vi "Get Common Path.vi"(9 "Root Path":path, 11 "Target Path":path) -> (2 "Paths Equal":bool, 3 "Relative Path":path)   [LabVIEW 2019, in "MD Generator.lvlib"]
uses:
  MD Generator.lvlib
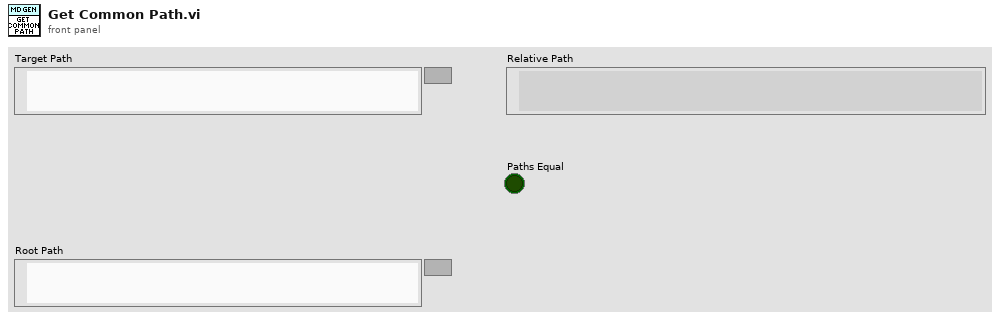
[diagram p1: front panel]
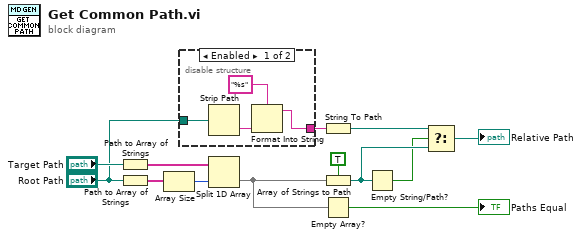
[diagram p0: block diagram]
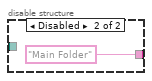
[diagram p2: hidden frame]
diagram:
  n1 = Path to Array of Strings(0:"Target Path") -> (2:w9:string[])  [unwired: 1 out]
  n2 = Path to Array of Strings(0:"Root Path") -> (2:w7:string[])  [unwired: 1 out]
  n3 = Array Size(array=w7) -> (size(s)=w4:i32)
  n4 = disable-structure shown="Enabled" {
    disable-tunnel: "Root Path" -> [w17 _]
    disable-tunnel: [w16 "Main Folder" ("format string")] -> w1
    frame Enabled {
      n5 = Strip Path(path=w17) -> (name=w15:string)  [unwired: 1 out]
      n6 = Format Into String(format string="%s", w15) -> (resulting string=w16:string)  [unwired: 2 in, 1 out]
    }
    frame Disabled {
    }
  }
  n7 = Split 1D Array(array=w9, index=w4) -> (second subarray=w11:string[])  [unwired: 1 out]
  n8 = String To Path(string=w1) -> (path=w6:path)
  n9 = Array of Strings to Path(0:w11, 1:TRUE ("relative")) -> (2:w5:path)
  n10 = Empty Array?(array=w11) -> (empty?=→"Paths Equal":bool)
  n11 = Empty String/Path?(string/path=w5) -> (empty?=w2:bool)
  n12 = Select(t=w6, s=w2, f=w5) -> (s? t:f=→"Relative Path":path)
